vi "4p1_HW_Task2_pipoat.vi"() -> ()   [LabVIEW 2016]
uses:
  <vilib>/express/express arith-compare/Formula/XNode/ExpressFormulaBlockNode.xnode
panel:
  out "Temperature":dbl
  in  "Resistance Associated (Ro)":dbl
  in  "Resistence of Thermistor at current temp (R)":dbl
  in  "Reference Temperature (To) (Celsius)":dbl
  in  "Thermal Property (B)":dbl
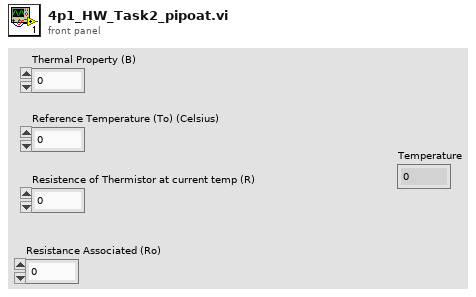
[diagram p1: front panel]
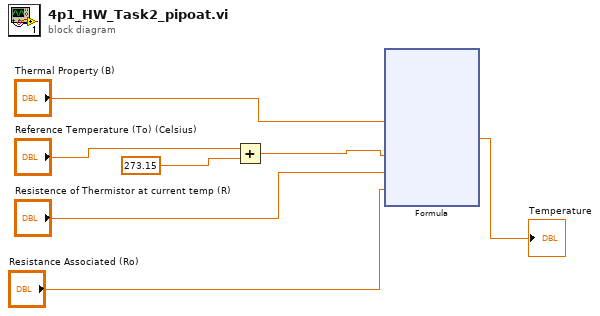
[diagram p0: block diagram]
diagram:
  n1 = Add(x="Reference Temperature (To) (Celsius)", y=273.15) -> (x+y=w1:dbl)
  n2 = xnode "Formula"("B"="Thermal Property (B)", "To"=w1, "R"="Resistence of Thermistor at current temp (R)", "Ro"="Resistance Associated (Ro)") -> ("Result"=→"Temperature":dbl)  [unwired: 1 in, 1 out]
